vi "main.vi"(8 "error in (no error)":errorcluster, 11 "builder settings":T1={"top level library"="plugin.lvlib", "plugin name"="", "plugin root folder"=path "D:/_repos/sandbox/Joao_Machado/Projects/LvAutomatedBuild/plugin", "version information"={"Product name"="", "Legal copyright"="", "Company name"="", "Internal name"="", "File description"=""}, "pre build vi path"=path "D:/_repos/sandbox/Joao_Machado/Projects/LvAutomatedBuild/builder/src/vis/pre_build_action_vi.vi", "post build vi path"=path "D:/_repos/sandbox/Joao_Machado/Projects/LvAutomatedBuild/builder/src/vis/post_build_action_vi.vi", "files to include"=["readme.txt", "about.txt", "image.png"], "version"={"Major"=1, "Minor"=2, "Fix"=3, "Build"=4}}) -> (0 "error out":errorcluster, 1 "Destinations":T4[](array[typedef]), 2 "root folder path":path=path "C:/Users/jmachado/AppData/Local/Temp/lvtemporary_222737.tmp", 3 "GeneratedFiles":path[](array[path]))   [LabVIEW 2024]
uses:
  <vilib>/AppBuilder/AB_API/common/AB_API Destination Data.ctl
  <vilib>/AppBuilder/AB_API/common/AB_API Destination Type.ctl
  typedefs/builder settings.ctl
  <vilib>/AppBuilder/AB_API/common/AB_API Version Information.ctl
  <vilib>/AppBuilder/AB_API/common/AB_API Version Number.ctl
  773ffeac-4f34-4c3b-abe1-b6f7e79432f6.vi
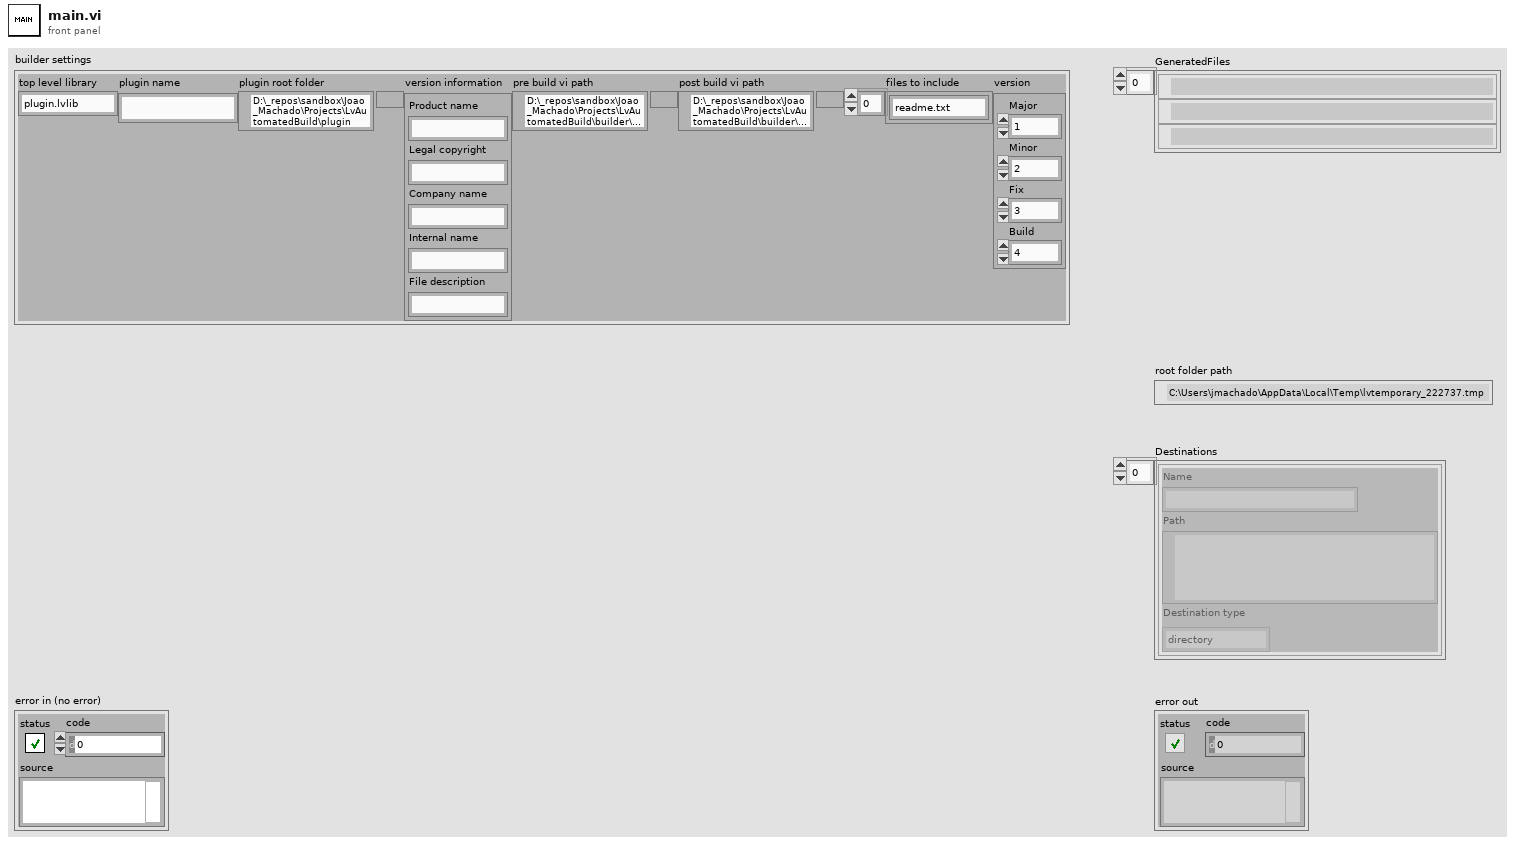
[diagram p1: front panel]
types:
  T1 = typedef "builder settings.ctl" = cluster{"top level library":string, "plugin name":string, "plugin root folder":path, "version information":T2, "pre build vi path":path, "post build vi path":path, "files to include":string[], "version":T3}
  T2 = typedef "AB_API Version Information.ctl" = cluster{"Product name":string, "Legal copyright":string, "Company name":string, "Internal name":string, "File description":string}
  T3 = typedef "AB_API Version Number.ctl" = cluster{"Major":u16, "Minor":u16, "Fix":u16, "Build":u16}
  T4 = typedef "AB_API Destination Data.ctl" = cluster{"Name":string, "Path":path, "Destination type":T5}
  T5 = typedef "AB_API Destination Type.ctl" = enum16{"directory", "directory (preserve hierarchy)", "LLB"}
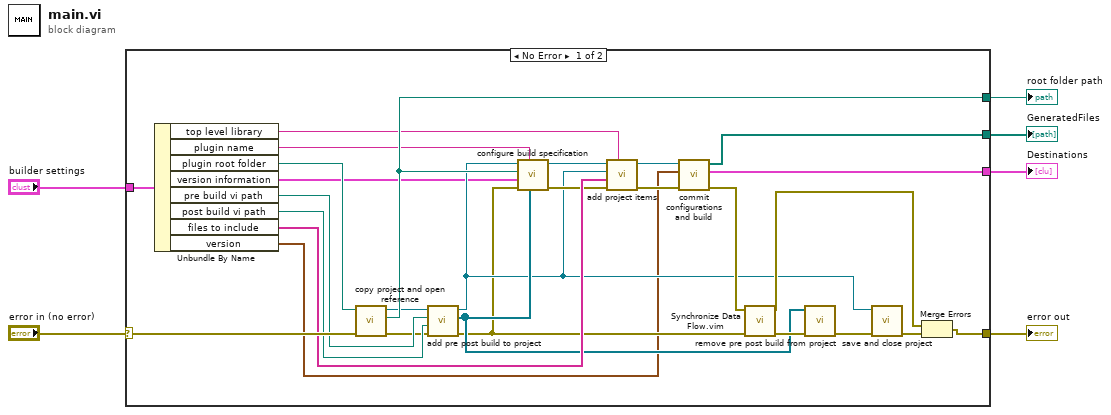
[diagram p0: block diagram]
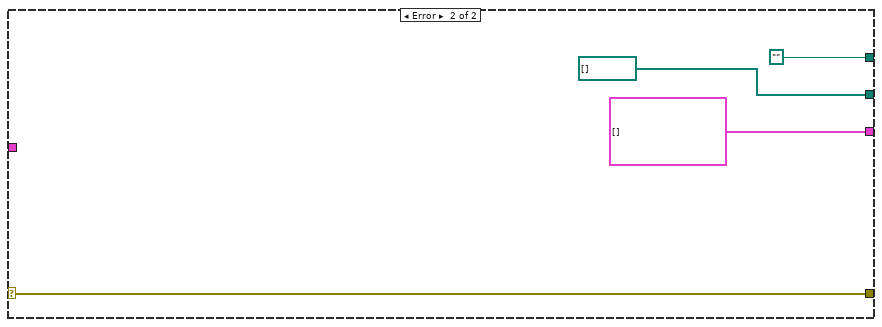
[diagram p2: hidden frame]
diagram:
  n1 = case shown="No Error" "error in (no error)" {
    selector: "error in (no error)" -> [w30 w38]
    tunnel: [w34 path ""] -> w6
    tunnel: [w33 path[] [] ("GeneratedFiles")] -> w1
    tunnel: [w32 T4[] [] ("Destinations")] -> w5
    tunnel: [w31 w38] -> w4
    tunnel: "builder settings" -> [w29 _]
    frame No Error {
      n2 = Unbundle By Name(w29) -> ("top level library"=w9:string, "plugin name"=w28:string, "plugin root folder"=w27:path, "version information"=w8:T2, "pre build vi path"=w26:path, "post build vi path"=w25:path, "files to include"=w24:string[], "version"=w7:T3)
      n3 = call "copy project and open reference.vi"("error in (no error)"=w30, "project_folder"=w27) -> ("error out"=w11:errorcluster, "root folder path"=w34:path, "Project Ref out"=w13:refnum<vi>)  [unwired: 7 in]
      n4 = call "add pre post build to project.vi"("error in (no error)"=w11, "post build action vi"=w25, "pre build action vi"=w26, "Project in"=w13) -> ("error out"=w10:errorcluster, "pre and post build refs"=w14:refnum<vi>[], "Project out"=w12:refnum<vi>)  [unwired: 5 in]
      n5 = call "configure build specification.vi"("pre and post build refs"=w14, "plugin name"=w28, "error in (no error)"=w10, "version information"=w8, "root folder path"=w34, "Project ref in"=w12) -> ("error out"=w20:errorcluster, "NI_AB_API_PPL out"=w19:refnum<class "NI_AB_API_PPL.lvclass">)  [unwired: 4 in]
      n6 = call "add project items.vi"("top level library"=w9, "error in (no error)"=w20, "items to add"=w24, "Project in"=w12, "NI_AB_API_PPL in"=w19) -> ("error out"=w21:errorcluster, "NI_AB_API_PPL out"=w22:refnum<class "NI_AB_API_PPL.lvclass">)  [unwired: 5 in]
      n7 = call "commit configurations and build.vi"("error in (no error)"=w21, "version"=w7, "NI_AB_API_PPL in"=w22) -> ("error out"=w18:errorcluster, "Destinations"=w32:T4[], "GeneratedFiles"=w33:path[])  [unwired: 6 in]
      n8 = call "Synchronize Data Flow.vim"("input 4"=w10, "input 1"=w18) -> ("output 4"=w17:errorcluster, "output 1"=w16:errorcluster)  [unwired: 2 in, 2 out]
      n9 = call "remove pre post build from project.vi"("error in (no error)"=w17, "pre and post build refs"=w14) -> ("error out"=w15:errorcluster)  [unwired: 9 in]
      n10 = call "save and close project.vi"("error in (no error)"=w15, "Project in"=w12) -> ("error out"=w23:errorcluster)  [unwired: 9 in]
      n11 = Merge Errors(w16, w23) -> (w31:errorcluster)
    }
    frame Error {
    }
  }
  "root folder path" <- w6
  "Destinations" <- w5
  "error out" <- w4
  "GeneratedFiles" <- w1
